vi "1A_BuildTriggerArray.vi"(0 "CBC Trigger Level":dbl, 1 "Load Resistance (Ohms)":dbl, 2 "Target Stim Current (Amps)":dbl, 3 "Krec Value":i32, 4 "Recovery Mode (T=Active)":bool) -> (5 "Pulse Triggers":T1(array[cluster]))   [LabVIEW 2010]
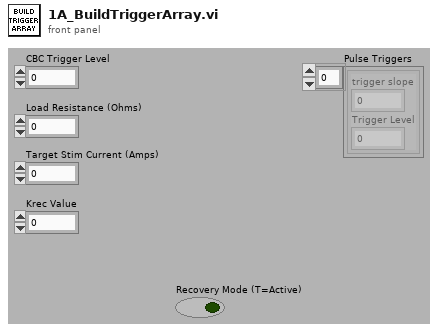
[diagram p1: front panel]
types:
  T1 = cluster{"trigger slope":u16, "Trigger Level":dbl}[]
  T2 = cluster{"trigger slope":u16, "Trigger Level":dbl}
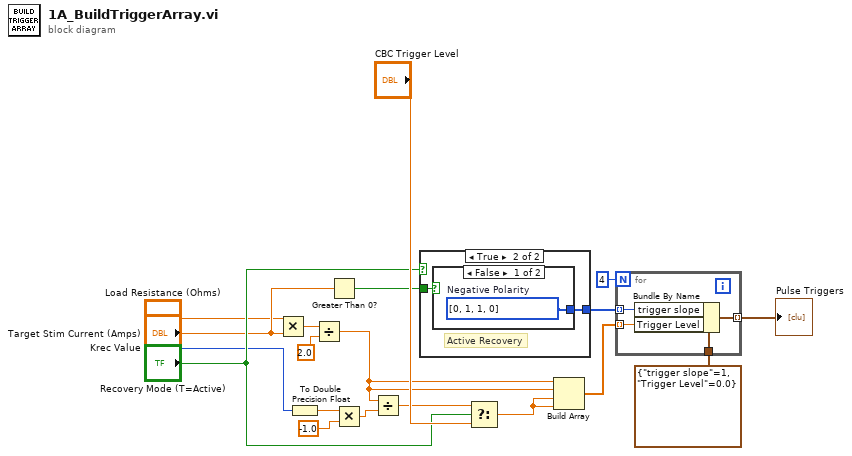
[diagram p0: block diagram]
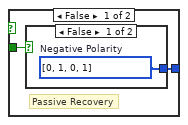
[diagram p2: hidden frame]
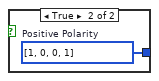
[diagram p3: hidden frame]
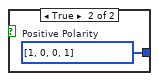
[diagram p4: hidden frame]
diagram:
  n1 = Multiply(x="Load Resistance (Ohms)", y="Target Stim Current (Amps)") -> (x*y=w4:dbl)
  n2 = To Double Precision Float(number="Krec Value") -> (double precision float=w12:dbl)
  n3 = Divide(x=w4, y=2.0) -> (x/y=w7:dbl)
  n4 = Greater Than 0?(x="Target Stim Current (Amps)") -> (x > 0?=w15:bool)
  n5 = Multiply(x=w12, y=-1.0) -> (x*y=w11:dbl)
  n6 = Divide(x=w7, y=w11) -> (x/y=w16:dbl)
  n7 = case shown="True" "Recovery Mode (T=Active)" {
    tunnel: [w20 w25] -> w3
    tunnel: w15 -> [w21 w24]
    frame False {
      # "Passive Recovery"
      n8 = case shown="False" w21 {
        tunnel: [w22 w23] -> w20
        frame False {
          w22 = u16[] [0, 1, 0, 1] items=["Falling Edge", "Rising Edge"]  # Negative Polarity
        }
        frame True {
          w23 = u16[] [1, 0, 0, 1] items=["Falling Edge", "Rising Edge"]  # Positive Polarity
        }
      }
    }
    frame True {
      # "Active Recovery"
      n9 = case shown="False" w24 {
        tunnel: [w26 w27] -> w25
        frame False {
          w26 = u16[] [0, 1, 1, 0] items=["Falling Edge", "Rising Edge"]  # Negative Polarity
        }
        frame True {
          w27 = u16[] [1, 0, 0, 1] items=["Falling Edge", "Rising Edge"]  # Positive Polarity
        }
      }
    }
  }
  n10 = Select(t=w16, s="Recovery Mode (T=Active)", f="CBC Trigger Level") -> (s? t:f=w17:dbl)
  n11 = Build Array(w7, w7, w17, w17) -> (w9:dbl[])
  n12 = for {
    N: 4 -> [_]
    tunnel: T2 {"trigger slope"=1, "Trigger Level"=0.0} -> [w31]
    tunnel: w3 -> [w30] mode=indexing
    tunnel: w9 -> [w29] mode=indexing
    tunnel: [w28] -> w10 mode=indexing
    n13 = Bundle By Name(cluster=w31, "trigger slope"=w30, "Trigger Level"=w29) -> (w28:T2)
  }
  "Pulse Triggers" <- w10
